vi "Flatten.vi"(8 "error in (no error)":errorcluster, 11 "Pulse Gen Scan in":refnum<class "Pulse Gen Scan.lvclass">) -> (0 "error out":errorcluster, 3 "Pulse Gen Scan out":refnum<class "Pulse Gen Scan.lvclass">)   [LabVIEW 2017, in "Pulse Gen Scan.lvclass"]
uses:
  Pulse Gen Scan.lvclass
  Pulse Gen Scan.lvclass/Pulse Gen Scan.ctl
  Global/File Locations.vi
  Scanner/Scanner.lvclass
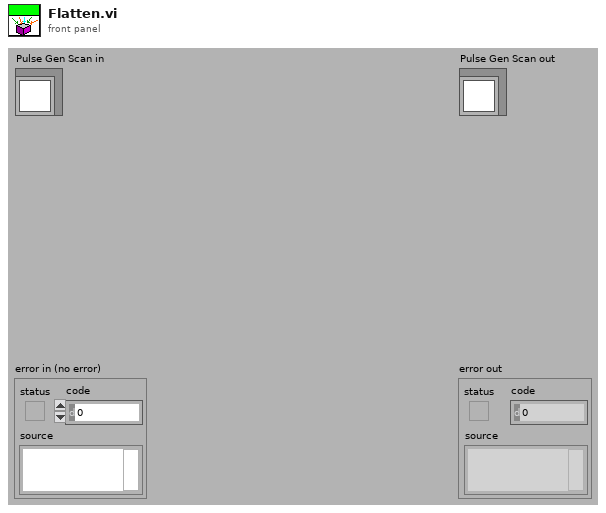
[diagram p1: front panel]
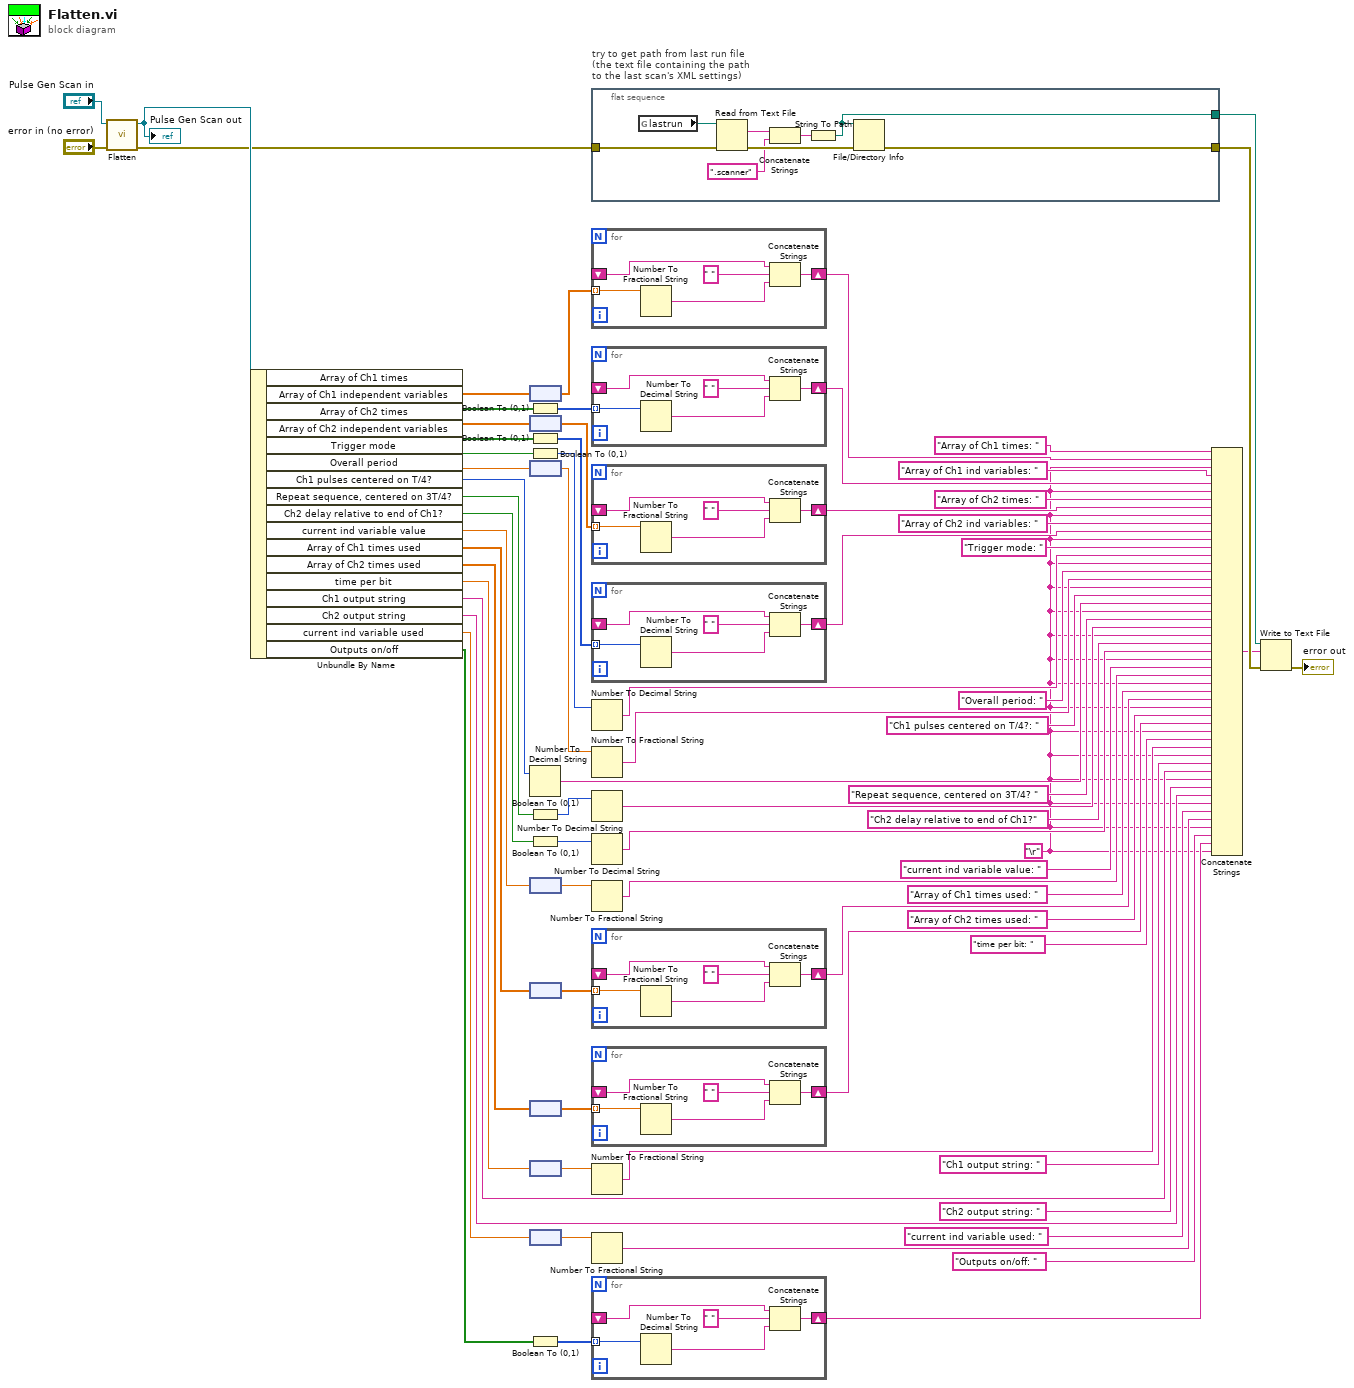
[diagram p0: block diagram]
diagram:
  w1 = "\r"
  n1 = call-parent "Flatten.vi"("error in (no error)"="error in (no error)", "Scanner in"="Pulse Gen Scan in") -> ("error out"=w69:errorcluster, "Scanner out"=w70:refnum<class "Pulse Gen Scan.lvclass">)  [unwired: 8 in]
  "Pulse Gen Scan out" <- w70
  n2 = Unbundle By Name(w70) -> ("Array of Ch1 times"=w64:dbl[unit][], "Array of Ch1 independent variables"=w57:bool[], "Array of Ch2 times"=w59:dbl[unit][], "Array of Ch2 independent variables"=w51:bool[], "Trigger mode"=w47:bool, "Overall period"=w43:dbl[unit], "Ch1 pulses centered on T/4?"=w39:enum32{"none", "first", "second"}, "Repeat sequence, centered on 3T/4?"=w35:bool, "Ch2 delay relative to end of Ch1?"=w34:bool, "current ind variable value"=w28:dbl[unit], "Array of Ch1 times used"=w23:dbl[unit][], "Array of Ch2 times used"=w22:dbl[unit][], "time per bit"=w15:dbl[unit], "Ch1 output string"=w12:string, "Ch2 output string"=w10:string, "current ind variable used"=w7:dbl[unit], "Outputs on/off"=w5:bool[])
  n3 = node(w64) -> (w63:dbl[])
  n4 = Boolean To (0,1)(Boolean=w57) -> (0, 1=w58:i16[])
  n5 = node(w59) -> (w60:dbl[])
  n6 = Boolean To (0,1)(Boolean=w51) -> (0, 1=w52:i16[])
  n7 = Boolean To (0,1)(Boolean=w47) -> (0, 1=w46:i16)
  n8 = node(w43) -> (w42:dbl)
  n9 = Number To Decimal String(number=w39) -> (decimal integer string=w38:string)  [unwired: 1 in]
  n10 = Boolean To (0,1)(Boolean=w35) -> (0, 1=w37:i16)
  n11 = Boolean To (0,1)(Boolean=w34) -> (0, 1=w36:i16)
  n12 = node(w28) -> (w27:dbl)
  n13 = node(w23) -> (w25:dbl[])
  n14 = node(w22) -> (w24:dbl[])
  n15 = node(w15) -> (w16:dbl)
  n16 = node(w7) -> (w8:dbl)
  n17 = Boolean To (0,1)(Boolean=w5) -> (0, 1=w4:i16[])
  n18 = flat-sequence "try to get path from last run file\n(the text file containing the path\nto the last scan's XML settings)" {
    tunnel: [w80] -> w67
    tunnel: [w77] -> w66
    tunnel: w69 -> [w76]
    frame #0 {
      n19 = global read "File Locations.vi" "lastrun"() -> (w79:path)
      n20 = Read from Text File(file (use dialog)=w79, error in=w76) -> (text=w75:string, error out=w78:errorcluster)  [unwired: 4 out]
      n21 = Concatenate Strings(w75, ".scanner") -> (w73:string)
      n22 = String To Path(string=w73) -> (path=w80:path)
      n23 = File/Directory Info(path=w80, error in=w78) -> (error out=w77:errorcluster)  [unwired: 6 out]
    }
  }
  n24 = for {
    tunnel: w63 -> [w85] mode=indexing
    shift-right: [w84] -> w62
    shift-left: _ -> [w83]
    n25 = Number To Fractional String(number=w85) -> (F-format string=w82:string)  [unwired: 3 in]
    n26 = Concatenate Strings(w83, " ", w82) -> (w84:string)
  }
  n27 = for {
    shift-right: [w90] -> w55
    shift-left: _ -> [w89]
    tunnel: w58 -> [w86] mode=indexing
    n28 = Number To Decimal String(number=w86) -> (decimal integer string=w87:string)  [unwired: 1 in]
    n29 = Concatenate Strings(w89, " ", w87) -> (w90:string)
  }
  n30 = for {
    tunnel: w60 -> [w95] mode=indexing
    shift-right: [w94] -> w53
    shift-left: _ -> [w93]
    n31 = Number To Fractional String(number=w95) -> (F-format string=w92:string)  [unwired: 3 in]
    n32 = Concatenate Strings(w93, " ", w92) -> (w94:string)
  }
  n33 = for {
    shift-right: [w100] -> w49
    shift-left: _ -> [w99]
    tunnel: w52 -> [w96] mode=indexing
    n34 = Number To Decimal String(number=w96) -> (decimal integer string=w97:string)  [unwired: 1 in]
    n35 = Concatenate Strings(w99, " ", w97) -> (w100:string)
  }
  n36 = Number To Decimal String(number=w46) -> (decimal integer string=w45:string)  [unwired: 1 in]
  n37 = Number To Fractional String(number=w42) -> (F-format string=w41:string)  [unwired: 3 in]
  n38 = Number To Decimal String(number=w37) -> (decimal integer string=w32:string)  [unwired: 1 in]
  n39 = Number To Decimal String(number=w36) -> (decimal integer string=w30:string)  [unwired: 1 in]
  n40 = Number To Fractional String(number=w27) -> (F-format string=w26:string)  [unwired: 3 in]
  n41 = for {
    tunnel: w25 -> [w105] mode=indexing
    shift-right: [w104] -> w20
    shift-left: _ -> [w103]
    n42 = Number To Fractional String(number=w105) -> (F-format string=w102:string)  [unwired: 3 in]
    n43 = Concatenate Strings(w103, " ", w102) -> (w104:string)
  }
  n44 = for {
    tunnel: w24 -> [w110] mode=indexing
    shift-right: [w109] -> w18
    shift-left: _ -> [w108]
    n45 = Number To Fractional String(number=w110) -> (F-format string=w107:string)  [unwired: 3 in]
    n46 = Concatenate Strings(w108, " ", w107) -> (w109:string)
  }
  n47 = Number To Fractional String(number=w16) -> (F-format string=w14:string)  [unwired: 3 in]
  n48 = Number To Fractional String(number=w8) -> (F-format string=w6:string)  [unwired: 3 in]
  n49 = for {
    shift-right: [w115] -> w2
    shift-left: _ -> [w114]
    tunnel: w4 -> [w111] mode=indexing
    n50 = Number To Decimal String(number=w111) -> (decimal integer string=w112:string)  [unwired: 1 in]
    n51 = Concatenate Strings(w114, " ", w112) -> (w115:string)
  }
  n52 = Concatenate Strings("Array of Ch1 times: ", w62, w1, "Array of Ch1 ind variables: ", w55, w1, "Array of Ch2 times: ", w53, w1, "Array of Ch2 ind variables: ", w49, w1, "Trigger mode: ", w45, w1, "Overall period: ", w41, w1, "Ch1 pulses centered on T/4?: ", w38, w1, "Repeat sequence, centered on 3T/4? ", w32, w1, "Ch2 delay relative to end of Ch1?", w30, w1, "current ind variable value: ", w26, w1, "Array of Ch1 times used: ", w20, w1, "Array of Ch2 times used: ", w18, w1, "time per bit: ", w14, w1, "Ch1 output string: ", w12, w1, "Ch2 output string: ", w10, w1, "current ind variable used: ", w6, w1, "Outputs on/off: ", w2, w1) -> (w65:string)
  n53 = Write to Text File(file (use dialog)=w67, text=w65, error in=w66) -> (error out=→"error out":errorcluster)  [unwired: 1 in, 2 out]
